vi "PrepDitheredImageNamesForPrinting.vi"(8 "error in (no error)":errorcluster, 9 "String":string, 10 "Head":i32, 11 "PPP_Dithered_Images":path) -> (0 "error out":errorcluster, 3 "appended path":path)   [LabVIEW 2022 SP3, in "TopLevel.lvclass"]
uses:
  TopLevel.lvclass
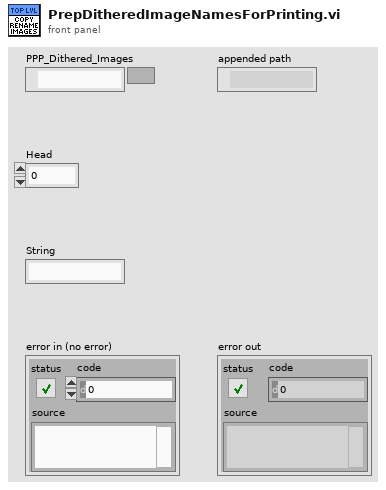
[diagram p1: front panel]
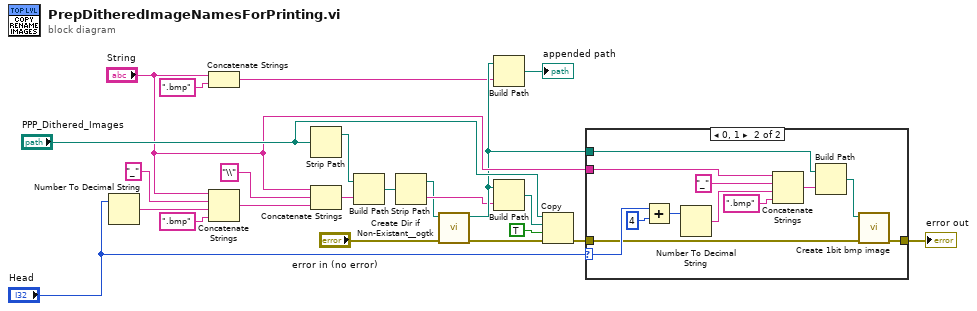
[diagram p0: block diagram]
diagram:
  n1 = Number To Decimal String(number="Head") -> (decimal integer string=w6:string)  [unwired: 1 in]
  n2 = Concatenate Strings("String", ".bmp" ("string")) -> (w14:string)
  n3 = Concatenate Strings("String", "_" ("string"), w6, ".bmp" ("string")) -> (w8:string)
  n4 = Strip Path(path="PPP_Dithered_Images") -> (stripped path=w1:path)  [unwired: 1 out]
  n5 = Concatenate Strings("String", "\\" ("string"), w8) -> (w3:string)
  n6 = Build Path(base path=w1, name or relative path=w3) -> (appended path=w11:path)
  n7 = Strip Path(path=w11) -> (stripped path=w12:path, name=w13:string)
  n8 = call <userlib>:"Create Dir if Non-Existant__ogtk.vi"("error in (no error)"="error in (no error)", "Directory Path"=w12) -> ("error out"=w9:errorcluster, "dup Directory Path"=w18:path)  [unwired: 7 in, 1 out]
  n9 = Build Path(base path=w18, name or relative path=w14) -> (appended path=→"appended path":path)
  n10 = Build Path(base path=w18, name or relative path=w13) -> (appended path=w16:path)
  n11 = Copy(8:w9, 9:TRUE ("overwrite (F)"), 10:w16, 11:"PPP_Dithered_Images") -> (0:w20:errorcluster)  [unwired: 1 in, 2 out]
  n12 = case shown="0, 1" "Head" {
    selector: "Head" -> [_ w36]
    tunnel: w18 -> [_ w34]
    tunnel: "String" -> [_ w30]
    tunnel: w20 -> [w24 w26]
    tunnel: [w24 w25] -> w23
    frame Default {
    }
    frame 0, 1 {
      n13 = Add(x=w36, y=4) -> (x+y=w29:i32)
      n14 = Number To Decimal String(number=w29) -> (decimal integer string=w32:string)  [unwired: 1 in]
      n15 = Concatenate Strings(w30, "_" ("string"), w32, ".bmp" ("string")) -> (w28:string)
      n16 = Build Path(base path=w34, name or relative path=w28) -> (appended path=w27:path)
      n17 = call "Create 1bit bmp image.vi"("error in (no error)"=w26, "path to BMP file"=w27) -> ("error out"=w25:errorcluster)  [unwired: 9 in]
    }
  }
  "error out" <- w23
